vi "test Loopback RT to RT with Start and Stop.vi"(8 "error in":errorcluster, 11 "TestCase in":refnum<class "Loopback.lvclass">) -> (0 "error out":errorcluster, 3 "TestCase out":refnum<class "Loopback.lvclass">)   [LabVIEW 2020, in "Loopback.lvclass"]
uses:
  Loopback.lvclass
  C:/dev/niveristand-custom-device-testing-tools/VeriStandTestCase/VeriStandTestCase.lvclass
  <vilib>/numeric/Random Number (Range) U64.vi
  485b7c2b-8320-4722-9ec7-d01f27c65546.vi
  1571aa8d-489e-4c94-925a-256c0ab49a50.vi
  a09b07c8-52ad-4e58-9957-78b331af32de.vi
  9426a44b-b3d4-42e7-bade-e6518c4f8208.vi
  <vilib>/numeric/sub_Random U32.vi
  <vilib>/NI VeriStand/Execution/Workspace/NI VeriStand - Set Multiple Channel Values.vi
  <vilib>/NI VeriStand/Execution/Workspace/NI VeriStand - Get Multiple Channel Values.vi
  <vilib>/NI VeriStand/Execution/Workspace/NI VeriStand - Set Single Channel Value.vi
  <vilib>/addons/_JKI Toolkits/VI Tester/TestCase.llb/TestCase.lvclass
  <vilib>/NI VeriStand/Execution/Workspace/NI_VS Workspace ExecutionAPI.lvlib
  C:/Program Files (x86)/National Instruments/LabVIEW 2020/vi.lib/addons/_JKI Toolkits/VI Tester/TestCase.llb/TestCase.lvclass
  C:/dev/niveristand-ballard-milStd1553-custom-device/Source/Custom Device Support/Tests/System/Loopback/Loopback.lvclass
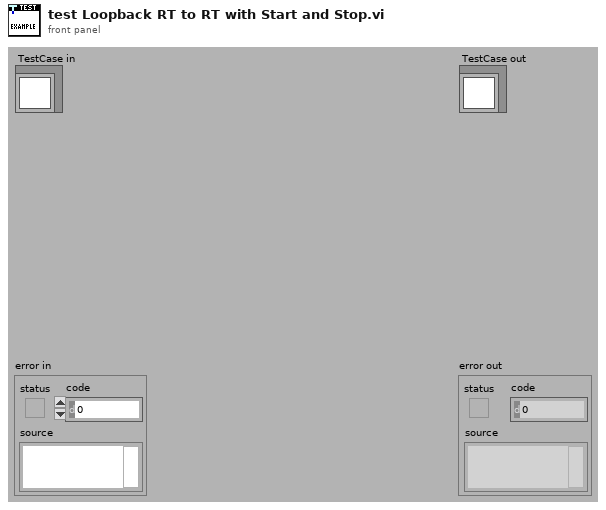
[diagram p1: front panel]
types:
  T1 = typedef "NI_VS Workspace ExecutionAPI.lvlib/WorkspaceAPI.ctl" = refnum<k24>
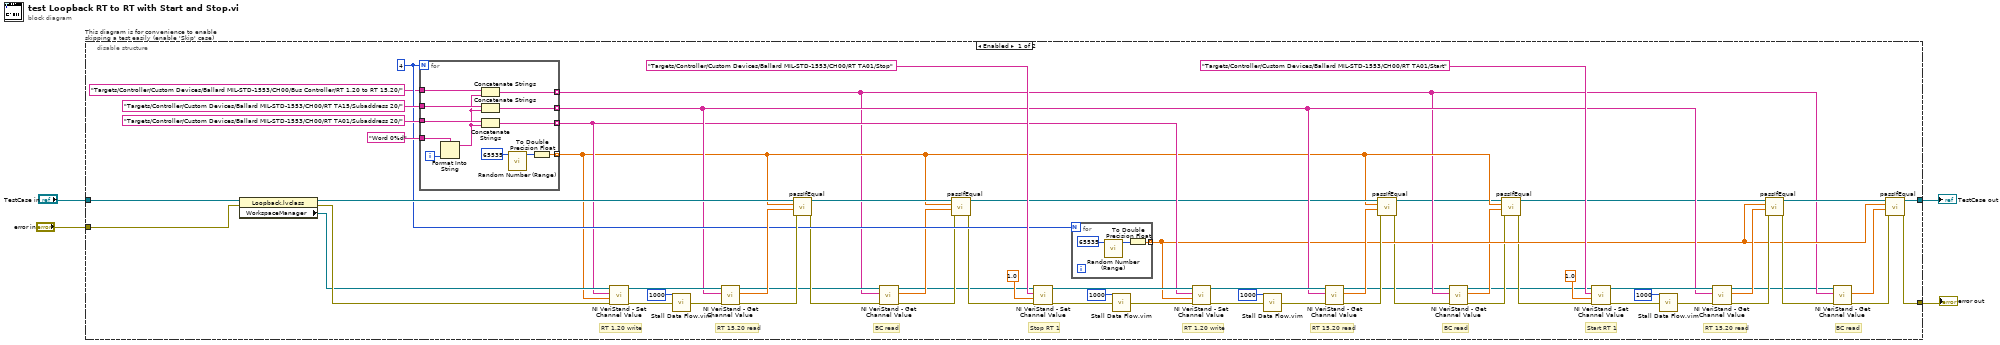
[diagram p0: block diagram]
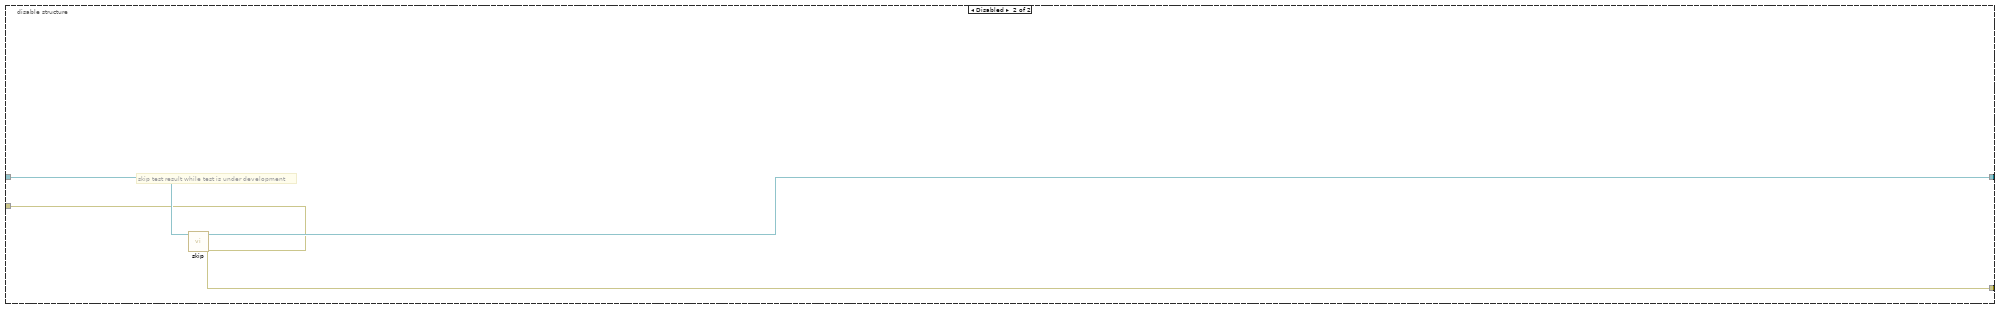
[diagram p2: hidden frame]
diagram:
  n1 = disable-structure "This diagram is for convenience to enable skipping a test easily (enable 'Skip' case)" shown="Enabled" {
    disable-tunnel: "TestCase in" -> [w59 w87]
    disable-tunnel: [w17 w85] -> w1
    disable-tunnel: [w18 w86] -> w3
    disable-tunnel: "error in" -> [w56 w84]
    frame Enabled {
      w34 = 4
      # "BC read"
      # "RT 15.20 read"
      # "BC read"
      # "RT 15.20 read"
      # "RT 1.20 write"
      # "BC read"
      # "RT 15.20 read"
      # "RT 1.20 write"
      # "Start RT 1"
      # "Stop RT 1"
      n2 = property class="Loopback.lvclass"(reference=w59, error in=w56) -> (reference out=w68:refnum<class "Loopback.lvclass">, error out=w63:errorcluster, "WorkspaceManager"=w61:T1)
      n3 = for {
        N: w34 -> [_]
        tunnel: "Targets/Controller/Custom Devices/Ballard MIL-STD-1553/CH00/RT TA01/Subaddress 20/" ("Channel") -> [w82]
        tunnel: [w83] -> w32 mode=indexing
        tunnel: "Targets/Controller/Custom Devices/Ballard MIL-STD-1553/CH00/RT TA15/Subaddress 20/" ("Channel") -> [w81]
        tunnel: [w80] -> w33 mode=indexing
        tunnel: "Word 0%d" -> [w78]
        tunnel: [w75] -> w12 mode=indexing
        tunnel: "Targets/Controller/Custom Devices/Ballard MIL-STD-1553/CH00/Bus Controller/RT 1.20 to RT 15.20/" ("Channel") -> [w74]
        tunnel: [w72] -> w11 mode=indexing
        i -> [w79]
        n4 = Format Into String(format string=w78, w79) -> (resulting string=w73:string)  [unwired: 2 in, 1 out]
        n5 = Concatenate Strings(w74, w73) -> (w72:string)
        n6 = Concatenate Strings(w81, w73) -> (w80:string)
        n7 = Concatenate Strings(w82, w73) -> (w83:string)
        n8 = call-poly <vilib>:"Random Number (Range).vi"("upper bound (100)"=u64 65535) -> ("number"=w77:u64)  [unwired: 10 in]
        n9 = To Double Precision Float(number=w77) -> (double precision float=w75:dbl)
      }
      n10 = call-poly <vilib>:"NI VeriStand - Set Channel Value.vi"("error in (no error)"=w63, "Values"=w12, "Channels"=w32, "WorkspaceManager in"=w61) -> ("error out"=w65:errorcluster, "WorkspaceManager out"=w67:T1)  [unwired: 6 in]
      n11 = call "Stall Data Flow.vim"("value in"=w65, "milliseconds to wait"=u32 1000) -> ("value out"=w66:errorcluster)  [unwired: 1 out]
      n12 = call-poly <vilib>:"NI VeriStand - Get Channel Value.vi"("error in (no error)"=w66, "Channels"=w33, "WorkspaceManager in"=w67) -> ("error out"=w62:errorcluster, "Values"=w60:dbl[], "WorkspaceManager out"=w24:T1)  [unwired: 6 in]
      n13 = call-dynamic "passIfEqual.vi"("error in (no error)"=w62, "y"=w60, "x"=w12, "TestCase in"=w68) -> ("error out"=w28:errorcluster, "TestCase out"=w26:refnum<class "Loopback.lvclass">)  [unwired: 6 in]
      n14 = call-poly <vilib>:"NI VeriStand - Get Channel Value.vi"("error in (no error)"=w28, "Channels"=w11, "WorkspaceManager in"=w24) -> ("error out"=w29:errorcluster, "Values"=w30:dbl[], "WorkspaceManager out"=w23:T1)  [unwired: 6 in]
      n15 = call-dynamic "passIfEqual.vi"("error in (no error)"=w29, "y"=w30, "x"=w12, "TestCase in"=w26) -> ("error out"=w27:errorcluster, "TestCase out"=w25:refnum<class "Loopback.lvclass">)  [unwired: 6 in]
      n16 = call-poly <vilib>:"NI VeriStand - Set Channel Value.vi"("error in (no error)"=w27, "Value"=1.0, "Channel"="Targets/Controller/Custom Devices/Ballard MIL-STD-1553/CH00/RT TA01/Stop", "WorkspaceManager in"=w23) -> ("error out"=w36:errorcluster, "WorkspaceManager out"=w52:T1)  [unwired: 6 in]
      n17 = for {
        N: w34 -> [_]
        tunnel: [w69] -> w16 mode=indexing
        n18 = call-poly <vilib>:"Random Number (Range).vi"("upper bound (100)"=u64 65535) -> ("number"=w70:u64)  [unwired: 10 in]
        n19 = To Double Precision Float(number=w70) -> (double precision float=w69:dbl)
      }
      n20 = call "Stall Data Flow.vim"("value in"=w36, "milliseconds to wait"=u32 1000) -> ("value out"=w35:errorcluster)  [unwired: 1 out]
      n21 = call-poly <vilib>:"NI VeriStand - Set Channel Value.vi"("error in (no error)"=w35, "Values"=w16, "Channels"=w32, "WorkspaceManager in"=w52) -> ("error out"=w39:errorcluster, "WorkspaceManager out"=w51:T1)  [unwired: 6 in]
      n22 = call "Stall Data Flow.vim"("value in"=w39, "milliseconds to wait"=u32 1000) -> ("value out"=w38:errorcluster)  [unwired: 1 out]
      n23 = call-poly <vilib>:"NI VeriStand - Get Channel Value.vi"("error in (no error)"=w38, "Channels"=w33, "WorkspaceManager in"=w51) -> ("error out"=w50:errorcluster, "Values"=w49:dbl[], "WorkspaceManager out"=w9:T1)  [unwired: 6 in]
      n24 = call-dynamic "passIfEqual.vi"("error in (no error)"=w50, "y"=w49, "x"=w12, "TestCase in"=w25) -> ("error out"=w13:errorcluster, "TestCase out"=w7:refnum<class "Loopback.lvclass">)  [unwired: 6 in]
      n25 = call-poly <vilib>:"NI VeriStand - Get Channel Value.vi"("error in (no error)"=w13, "Channels"=w11, "WorkspaceManager in"=w9) -> ("error out"=w14:errorcluster, "Values"=w15:dbl[], "WorkspaceManager out"=w8:T1)  [unwired: 6 in]
      n26 = call-dynamic "passIfEqual.vi"("error in (no error)"=w14, "y"=w15, "x"=w12, "TestCase in"=w7) -> ("error out"=w10:errorcluster, "TestCase out"=w6:refnum<class "Loopback.lvclass">)  [unwired: 6 in]
      n27 = call-poly <vilib>:"NI VeriStand - Set Channel Value.vi"("error in (no error)"=w10, "Value"=1.0, "Channel"="Targets/Controller/Custom Devices/Ballard MIL-STD-1553/CH00/RT TA01/Start", "WorkspaceManager in"=w8) -> ("error out"=w45:errorcluster, "WorkspaceManager out"=w41:T1)  [unwired: 6 in]
      n28 = call "Stall Data Flow.vim"("value in"=w45, "milliseconds to wait"=u32 1000) -> ("value out"=w42:errorcluster)  [unwired: 1 out]
      n29 = call-poly <vilib>:"NI VeriStand - Get Channel Value.vi"("error in (no error)"=w42, "Channels"=w33, "WorkspaceManager in"=w41) -> ("error out"=w43:errorcluster, "Values"=w44:dbl[], "WorkspaceManager out"=w5:T1)  [unwired: 6 in]
      n30 = call-dynamic "passIfEqual.vi"("error in (no error)"=w43, "y"=w44, "x"=w16, "TestCase in"=w6) -> ("error out"=w19:errorcluster, "TestCase out"=w20:refnum<class "Loopback.lvclass">)  [unwired: 6 in]
      n31 = call-poly <vilib>:"NI VeriStand - Get Channel Value.vi"("error in (no error)"=w19, "Channels"=w11, "WorkspaceManager in"=w5) -> ("error out"=w22:errorcluster, "Values"=w21:dbl[])  [unwired: 6 in, 1 out]
      n32 = call-dynamic "passIfEqual.vi"("error in (no error)"=w22, "y"=w21, "x"=w16, "TestCase in"=w20) -> ("error out"=w18:errorcluster, "TestCase out"=w17:refnum<class "Loopback.lvclass">)  [unwired: 6 in]
    }
    frame Disabled {
      # "skip test result while test is under development"
      n33 = call <vilib>:"skip.vi"("error in (no error)"=w84, "TestCase in"=w87) -> ("error out"=w86:errorcluster, "TestCase out"=w85:refnum<class "Loopback.lvclass">)  [unwired: 8 in]
    }
  }
  "error out" <- w3
  "TestCase out" <- w1
